vi "6.Bounce Window_ERROR.vi"(11 "MSG In":string) -> (3 "Error Action Out":T1)   [LabVIEW 2015]
uses:
  0.Main_Control/Control_Bounce Window_Main_FGV_Error Action.ctl
  <vilib>/Utility/miscctls.llb/LVPointTypeDef.ctl
panel:
  in  "確認":bool
  in  "Error Action":T1
  out "MSG Out":string
  # "錯誤訊息"
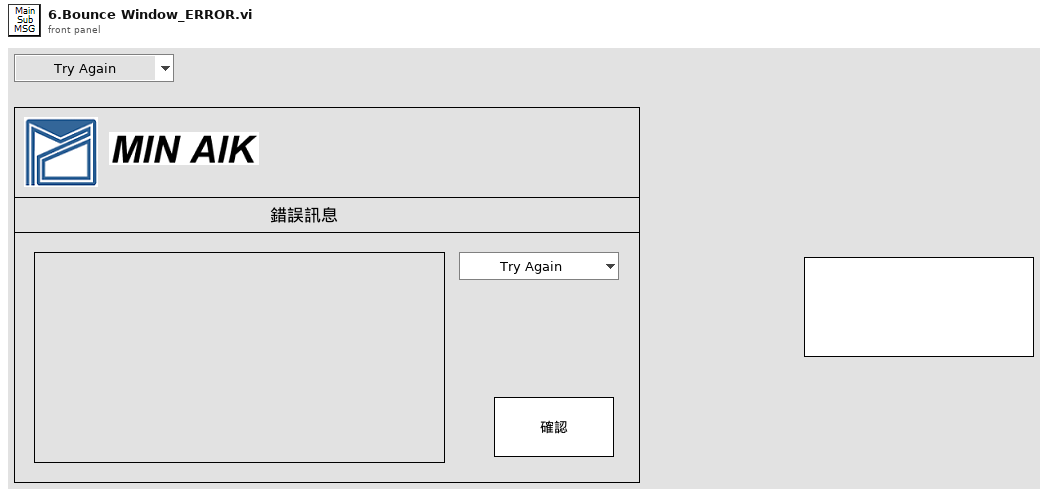
[diagram p1: front panel]
types:
  T1 = typedef "Control_Bounce Window_Main_FGV_Error Action.ctl" = enum16{"Try Again", "Stop"}
  T2 = typedef "LVPointTypeDef.ctl" = cluster{"Horizontal":i16, "Vertical":i16}
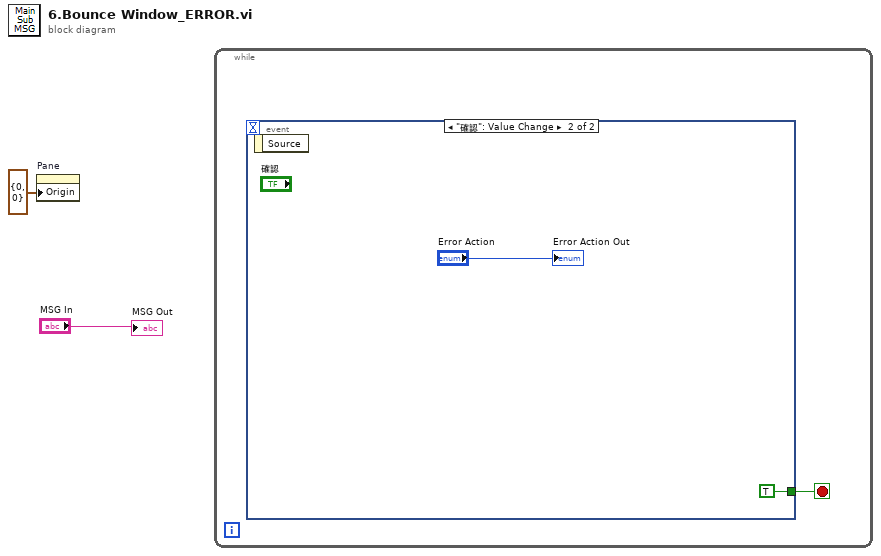
[diagram p0: block diagram]
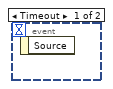
[diagram p2: hidden frame]
diagram:
  n1 = property on="Pane" class="Pane"("Origin"=T2 {"Horizontal"=0, "Vertical"=0}) -> ()  [unwired: 2 in, 2 out]
  n2 = while {
    stop <- w3 stop-if-true
    n3 = event shown="[1] \"確認\": Value Change" {
      selector: _ -> [_ _]
      dyn-events: _ -> [_ _]
      timeout: _ -> [_ _]
      tunnel: [_ TRUE] -> w3
      event Timeout {
        n4 = event-data() -> ()  [unwired: 1 in, 1 out]
      }
      event "確認": Value Change {
        n5 = event-data() -> ()  [unwired: 1 in, 1 out]
        "Error Action Out" <- "Error Action"
      }
    }
  }
  "MSG Out" <- "MSG In"
